vi "Test Method Template 1.vi"(11 "Test Case In":refnum<class "Test Config From EXCEL.lvclass">) -> (0 "error out":errorcluster, 3 "Test Case Out":refnum<class "Test Config From EXCEL.lvclass">)   [LabVIEW 2024, in "Test Config From EXCEL.lvclass"]
uses:
  Test Config From EXCEL.lvclass
  C:/Program Files/National Instruments/LabVIEW 2025/vi.lib/Astemes/LUnit/Test Case.lvclass
  Config from EXCEL/Config from EXCEL.lvclass
  <vilib>/Astemes/LUnit/Test Case.lvclass/Test Case.ctl
  Test Config From EXCEL.lvclass/Test Config From EXCEL.ctl
  <vilib>/Astemes/LUnit/Test Case.lvclass
  C:/Program Files/National Instruments/LabVIEW 2025/vi.lib/Astemes/LUnit/LUnit Runnable.lvclass
  D:/git/HAL/Source/Test Config From EXCEL/Test Config From EXCEL.lvclass
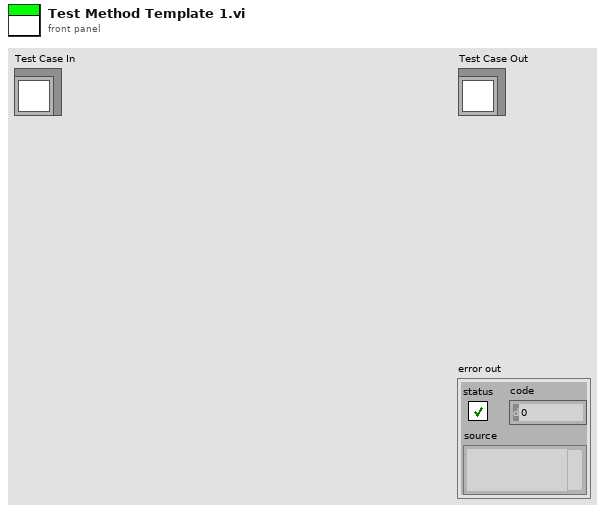
[diagram p1: front panel]
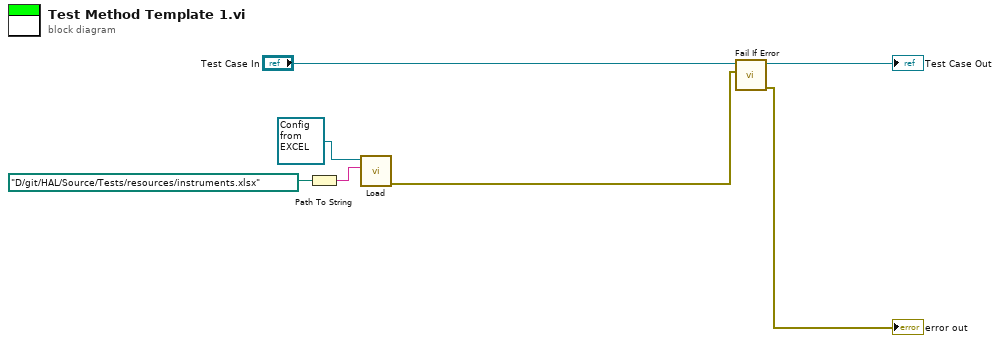
[diagram p0: block diagram]
diagram:
  n1 = Path To String(path=path "D:/git/HAL/Source/Tests/resources/instruments.xlsx") -> (string=w2:string)
  n2 = call-dynamic "Load.vi"("Source"=w2, "Config from EXCEL in"=refnum<class "Config from EXCEL.lvclass"> refnum ("Config from EXCEL.lvclass")) -> ("error out"=w1:errorcluster)  [unwired: 8 in, 1 out]
  n3 = call <vilib>:"Fail If Error.vi"("Assert error"=w1, "LUnit Test Case In"="Test Case In") -> ("error out"=→"error out":errorcluster, "LUnit Test Case Out"=→"Test Case Out":refnum<class "Test Config From EXCEL.lvclass">)  [unwired: 8 in]
